vi "data_handler.vi"(5 "字符串":string) -> (0 "X":string, 1 "Y":string, 2 "Z":string, 3 "Speed":string, 4 "Command":string)   [LabVIEW 2018]
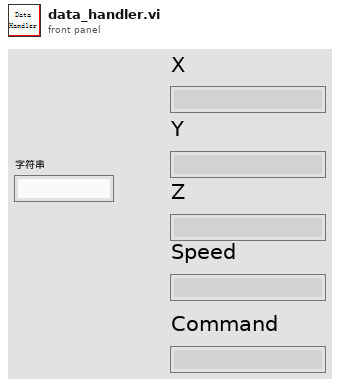
[diagram p1: front panel]
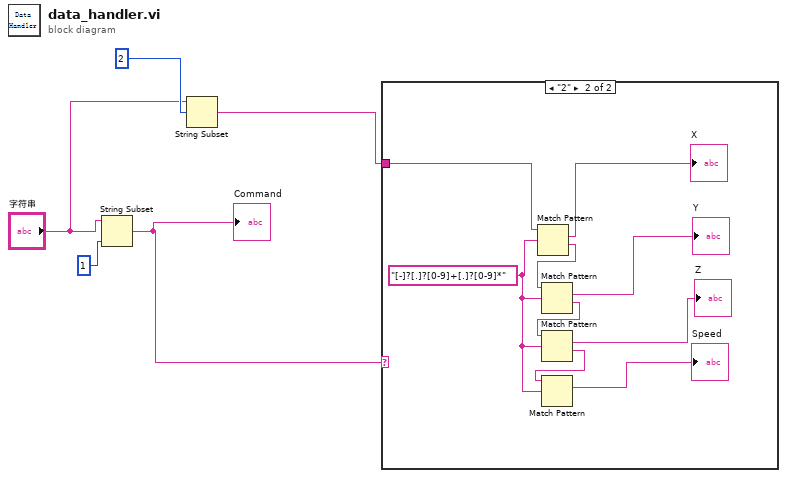
[diagram p0: block diagram]
diagram:
  n1 = String Subset(string="字符串", length (rest)=1) -> (substring=w4:string)  [unwired: 1 in]
  "Command" <- w4
  n2 = String Subset(string="字符串", offset (0)=2) -> (substring=w1:string)  [unwired: 1 in]
  n3 = case shown="\"2\"" w4 {
    tunnel: w1 -> [_ w14]
    frame "1", Default {
    }
    frame "2" {
      w6 = "[-]?[.]?[0-9]+[.]?[0-9]*"
      n4 = Match Pattern(string=w14, regular expression=w6) -> (match substring=→"X":string, after substring=w12:string)  [unwired: 1 in, 2 out]
      n5 = Match Pattern(string=w12, regular expression=w6) -> (match substring=→"Y":string, after substring=w11:string)  [unwired: 1 in, 2 out]
      n6 = Match Pattern(string=w11, regular expression=w6) -> (match substring=→"Z":string, after substring=w7:string)  [unwired: 1 in, 2 out]
      n7 = Match Pattern(string=w7, regular expression=w6) -> (match substring=→"Speed":string)  [unwired: 1 in, 3 out]
    }
  }
